vi "SET Enqueuers Array 2 Dispatch Message.vi"(8 "error in (no error)":errorcluster, 10 "Enqueuers Array":refnum<class "Message Enqueuer.lvclass">[](array[class]), 11 "Child_5_Class in":refnum<class "Error_Emgime_Class.lvclass">) -> (0 "error out":errorcluster, 3 "Child_5_Class out":refnum<class "Error_Emgime_Class.lvclass">)   [LabVIEW 2023, in "Error_Engine_Actor.lvlib" / "Error_Emgime_Class.lvclass"]
uses:
  Error_Emgime_Class.lvclass
  <vilib>/ActorFramework/Message Enqueuer/Message Enqueuer.lvclass
  Abstraction_Interface_Class/Abstraction_Interface_Class.lvclass
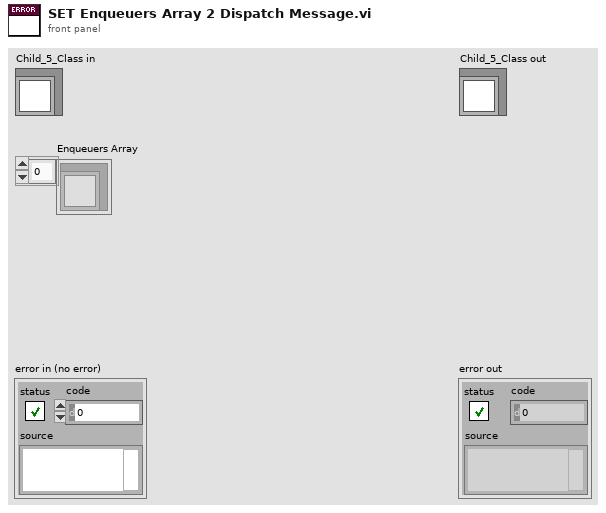
[diagram p1: front panel]
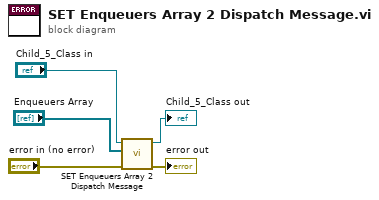
[diagram p0: block diagram]
diagram:
  n1 = call-parent "SET Enqueuers Array 2 Dispatch Message.vi"("error in (no error)"="error in (no error)", "Enqueuers Array"="Enqueuers Array", "Interface_Class in"="Child_5_Class in") -> ("error out"=→"error out":errorcluster, "Interface_Class out"=→"Child_5_Class out":refnum<class "Error_Emgime_Class.lvclass">)  [unwired: 7 in]
